vi "generate_step_array.vi"(1 "Max Potential (V)":dbl, 2 "Current Potential (V)":dbl, 3 "Target Potential (V)":dbl) -> (0 "Step Array":dbl[](array[numeric]))   [LabVIEW 2019]
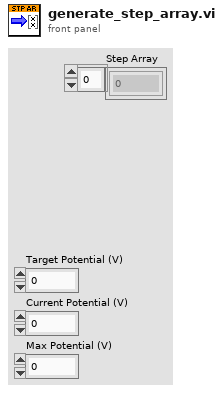
[diagram p1: front panel]
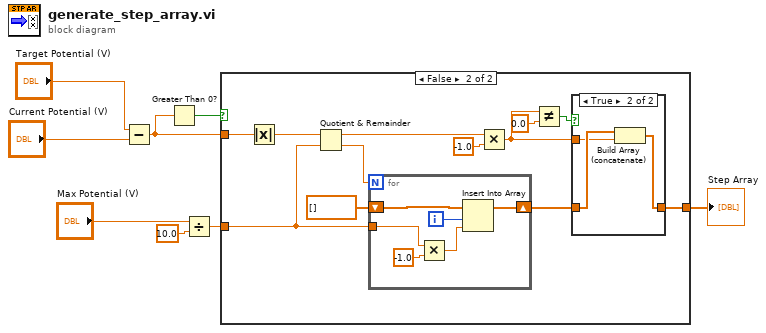
[diagram p0: block diagram]
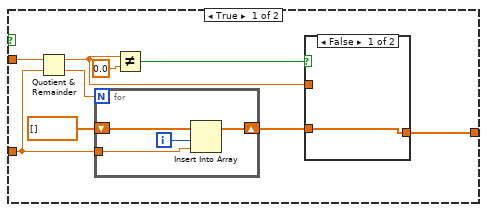
[diagram p2: hidden frame]
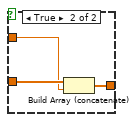
[diagram p3: hidden frame]
diagram:
  n1 = Subtract(x="Target Potential (V)", y="Current Potential (V)") -> (x-y=w2:dbl)
  n2 = Greater Than 0?(x=w2) -> (x > 0?=w3:bool)
  n3 = Divide(x="Max Potential (V)", y=10.0) -> (x/y=w6:dbl)
  n4 = case shown="False" w3 {
    tunnel: w6 -> [w16 w36]
    tunnel: w2 -> [w9 w30]
    tunnel: [w10 w31] -> w1
    frame True {
      n5 = Quotient & Remainder(x=w9, y=w16) -> (x-y*floor(x/y)=w11:dbl, floor(x/y)=w17:dbl)
      n6 = for {
        N: w17 -> [_]
        shift-right: [w24] -> w12
        shift-left: dbl[] [] -> [w25]
        tunnel: w16 -> [w22]
        i -> [w23]
        n7 = Insert Into Array(array=w25, index=w23, new element=w22) -> (w24:dbl[])
      }
      n8 = Not Equal?(x=w11, y=0.0) -> (x != y?=w14:bool)
      n9 = case shown="False" w14 {
        tunnel: w12 -> [w18 w21]
        tunnel: w11 -> [_ w20]
        tunnel: [w18 w19] -> w10
        frame False {
        }
        frame True {
          n10 = Build Array (concatenate)(w21, w20) -> (w19:dbl[])
        }
      }
    }
    frame False {
      n11 = Absolute Value(x=w30) -> (abs(x)=w29:dbl)
      n12 = Quotient & Remainder(x=w29, y=w36) -> (x-y*floor(x/y)=w28:dbl, floor(x/y)=w37:dbl)
      n13 = for {
        N: w37 -> [_]
        shift-right: [w46] -> w32
        shift-left: dbl[] [] -> [w47]
        tunnel: w36 -> [w43]
        i -> [w45]
        n14 = Multiply(x=w43, y=-1.0) -> (x*y=w42:dbl)
        n15 = Insert Into Array(array=w47, index=w45, new element=w42) -> (w46:dbl[])
      }
      n16 = Multiply(x=w28, y=-1.0) -> (x*y=w26:dbl)
      n17 = Not Equal?(x=w26, y=0.0) -> (x != y?=w34:bool)
      n18 = case shown="True" w34 {
        tunnel: w32 -> [w38 w41]
        tunnel: w26 -> [_ w40]
        tunnel: [w38 w39] -> w31
        frame False {
        }
        frame True {
          n19 = Build Array (concatenate)(w41, w40) -> (w39:dbl[])
        }
      }
    }
  }
  "Step Array" <- w1
